vi "File to TDMS.vi"(8 "error in (no error)":errorcluster, 9 "Single File? [T]":bool=TRUE, 10 "Path":path, 11 "Conversion.lvclass":refnum<class "Conversion.lvclass">) -> (0 "error out":errorcluster, 1 "Not Equal?":bool, 3 "Conversion.lvclass out":refnum<class "Conversion.lvclass">)   [LabVIEW 2020, in "Conversion.lvclass"]
uses:
  Conversion.lvclass
  Data/Data.lvclass
  Data/Typedefs/File Type--enum.ctl
  Data/Typedefs/Operation--enum.ctl
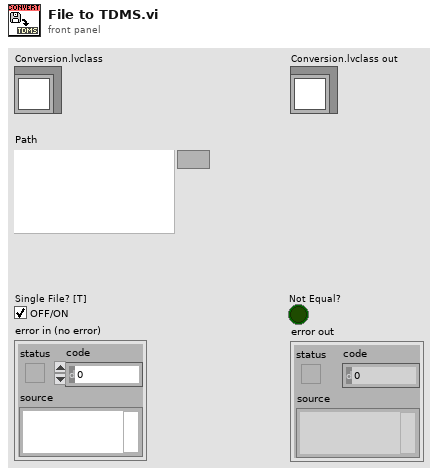
[diagram p1: front panel]
types:
  T1 = typedef "Data.lvclass/File Type--enum.ctl" = enum16{"DAT", "ITX", "HDF5", "TDMS", "VI", "PGSQL"}
  T2 = typedef "Data.lvclass/Operation--enum.ctl" = enum16{"Read", "Write", "Write + Append"}
  T3 = typedef "Data.lvclass/Dictionary--cluster.ctl" = cluster{"key":string, "value":variant}
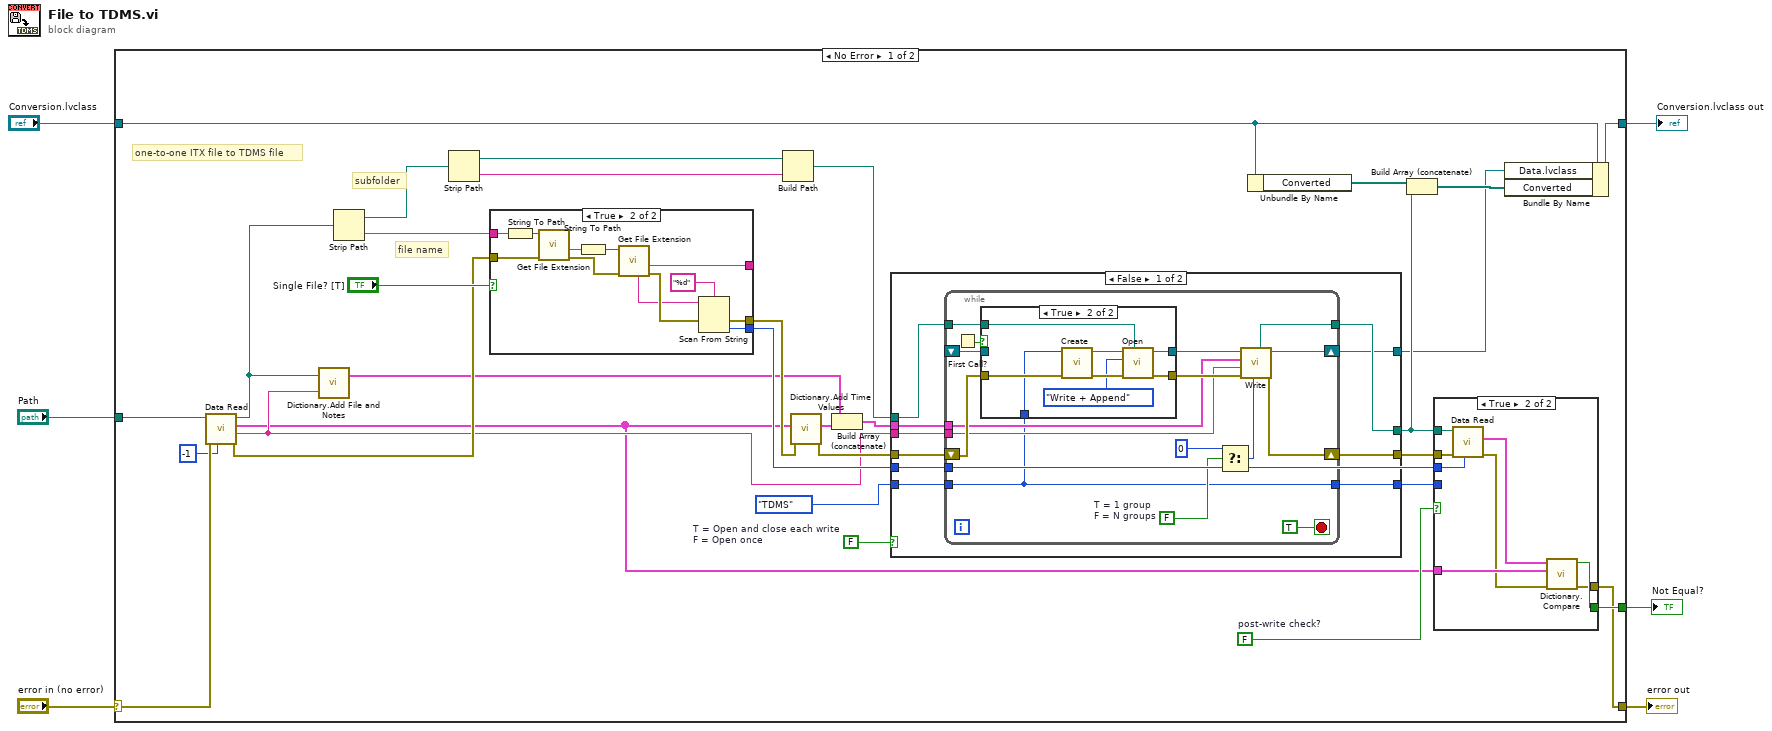
[diagram p0: block diagram]
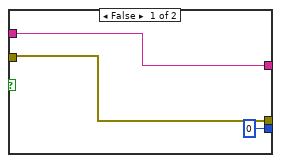
[diagram p3: hidden frame]
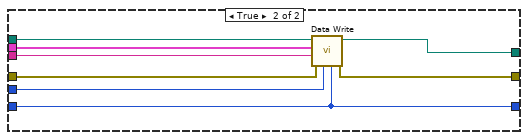
[diagram p5: hidden frame]
diagram:
  n1 = case shown="No Error" "error in (no error)" {
    selector: "error in (no error)" -> [w37 w108]
    tunnel: [w34 w108] -> w5
    tunnel: "Path" -> [w38 _]
    tunnel: [w35 _] -> w3
    tunnel: [w14 _] -> w2
    tunnel: "Conversion.lvclass" -> [w12 _]
    frame No Error {
      w19 = FALSE  # post-write check?
      w30 = FALSE  # T = Open and close each write F = Open once
      # "file name"
      # "subfolder"
      # "one-to-one ITX file to TDMS file"
      n2 = call "Data Read.vi"("Append Index"=-1, "error in (no error)"=w37, "path"=w38) -> ("error out"=w29:errorcluster, "Notes"=w24:string, "Data (Dictionary)"=w13:T3[], "path out"=w25:path)  [unwired: 5 in]
      n3 = call "Dictionary.Add File and Notes.vi"("Notes"=w24, "Path"=w25) -> ("Dictionary"=w20:T3[])  [unwired: 1 in]
      n4 = Strip Path(path=w25) -> (stripped path=w18:path, name=w16:string)
      n5 = Strip Path(path=w18) -> (stripped path=w17:path, name=w15:string)
      n6 = case shown="True" "Single File? [T]" {
        tunnel: w29 -> [w48 w62]
        tunnel: w16 -> [w50 w59]
        tunnel: [w50 w51] -> _
        tunnel: [0 w52] -> w31
        tunnel: [w48 w57] -> w27
        frame False {
        }
        frame True {
          n7 = String To Path(string=w59) -> (path=w58:path)
          n8 = call <vilib>:"Get File Extension.vi"("error in (no error)"=w62, "file"=w58) -> ("error out"=w56:errorcluster, "filename without extension"=w60:string)  [unwired: 8 out]
          n9 = String To Path(string=w60) -> (path=w61:path)
          n10 = call <vilib>:"Get File Extension.vi"("error in (no error)"=w56, "file"=w61) -> ("error out"=w54:errorcluster, "filename without extension"=w51:string, "unmodified file extension"=w53:string)  [unwired: 7 out]
          n11 = Scan From String(format string="%d", input string=w53, error in=w54) -> (error out=w57:errorcluster, output 1=w52:i32)  [unwired: 2 in, 2 out]
        }
      }
      n12 = Build Path(base path=w17, name or relative path=w15) -> (appended path=w33:path)
      n13 = call "Dictionary.Add Time Values.vi"("error in (no error)"=w27, "Data (Dictionary)"=w13) -> ("error out"=w26:errorcluster, "Dictionary"=w28:T3[])  [unwired: 8 in]
      n14 = Build Array (concatenate)(w20, w28) -> (w21:T3[])
      n15 = case shown="False" w30 {
        tunnel: w24 -> [w69 w107]
        tunnel: [w65 w106] -> w9
        tunnel: [w71 w105] -> w36
        tunnel: w21 -> [w70 w104]
        tunnel: w26 -> [w72 w103]
        tunnel: w33 -> [w66 w102]
        tunnel: [w67 w100] -> w23
        tunnel: w31 -> [w68 w101]
        tunnel: [w64 _] -> w8
        tunnel: File_Type--enum."TDMS" ("File Type") -> [w63 w100]
        frame False {
          n16 = while {
            tunnel: w70 -> [w85]
            tunnel: w69 -> [w84]
            tunnel: w68 -> [w76]
            tunnel: [w73] -> w67
            tunnel: w66 -> [w83]
            shift-right: [w86] -> w71
            shift-left: w72 -> [w87]
            shift-right: [w82] -> w64
            shift-left: _ -> [w80]
            tunnel: [w78] -> w65
            tunnel: w63 -> [w73]
            stop <- TRUE stop-if-true
            w75 = FALSE  # T = 1 group F = N groups
            n17 = First Call?() -> (First Call?: T/F=w81:bool)
            n18 = case shown="True" w81 {
              tunnel: [w90 w99] -> w89
              tunnel: [w91 w98] -> w88
              tunnel: w87 -> [w90 w95]
              tunnel: w73 -> [_ w94]
              tunnel: w83 -> [_ w93]
              tunnel: w80 -> [w91 _]
              frame False {
              }
              frame True {
                n19 = call "Create.vi"("error in (no error)"=w95, "File Type"=w94) -> ("error out"=w96:errorcluster, "Data out"=w97:refnum<class "Data.lvclass">)  [unwired: 8 in]
                n20 = call-dynamic "Open.vi"("Path"=w93, "error in (no error)"=w96, "Operation"=Operation--enum."Write + Append", "Data in"=w97) -> ("error out"=w99:errorcluster, "Data out"=w98:refnum<class "Data.lvclass">)  [unwired: 6 in]
              }
            }
            n21 = Select(t=0 ("Append Index"), s=w75, f=w76) -> (s? t:f=w74:i32)
            n22 = call-dynamic "Write.vi"("Append Index"=w74, "error in (no error)"=w89, "Notes"=w84, "Data (Dictionary)"=w85, "Data in"=w88) -> ("error out"=w86:errorcluster, "Data out"=w82:refnum<class "Data.lvclass">, "Path out"=w78:path)  [unwired: 4 in]
          }
        }
        frame True {
          n23 = call "Data Write.vi"("File Type"=w100, "Append Index"=w101, "error in (no error)"=w103, "Notes"=w107, "Data (Dictionary)"=w104, "path"=w102) -> ("error out"=w105:errorcluster, "path out"=w106:path)  [unwired: 4 in]
        }
      }
      n24 = Unbundle By Name(w12) -> ("Converted"=w11:path[])
      n25 = Build Array (concatenate)(w11, w9) -> (w10:path[])
      n26 = case shown="True" w19 {
        tunnel: w9 -> [_ w47]
        tunnel: w36 -> [w39 w46]
        tunnel: [_ w45] -> w35
        tunnel: [w39 w44] -> w34
        tunnel: w31 -> [_ w43]
        tunnel: w13 -> [_ w42]
        tunnel: w23 -> [_ _]
        frame False {
        }
        frame True {
          n27 = call "Data Read.vi"("Append Index"=w43, "error in (no error)"=w46, "path"=w47) -> ("error out"=w41:errorcluster, "Data (Dictionary)"=w40:T3[])  [unwired: 5 in, 2 out]
          n28 = call "Dictionary.Compare.vi"("error in (no error)"=w41, "Original Data (Dictionary)"=w42, "Converted Data (Dictionary)"=w40) -> ("error out"=w44:errorcluster, "Not Equal?"=w45:bool)  [unwired: 7 in]
        }
      }
      n29 = Bundle By Name(cluster=w12, "Data.lvclass"=w8, "Converted"=w10) -> (w14:refnum<class "Conversion.lvclass">)
    }
    frame Error {
    }
  }
  "error out" <- w5
  "Not Equal?" <- w3
  "Conversion.lvclass out" <- w2
